vi "VI, Grow Panel Height to Control.vi"(5 "margin (20)":i32=20, 6 "error in":errorcluster, 8 "Ctl ref":refnum<vi>, 9 "VI ref":refnum<vi>) -> (0 "error out":errorcluster, 2 "Ctl ref dup":refnum<vi>, 3 "VI ref dup":refnum<vi>)   [LabVIEW 2010]
doc: "This function increases a panels width to display a control."
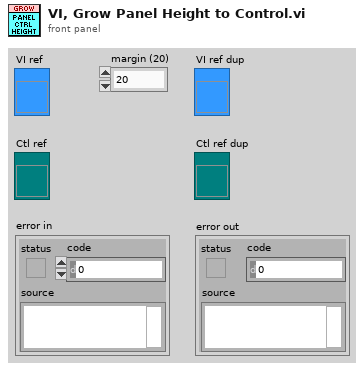
[diagram p1: front panel]
types:
  T1 = typedef "LVRectTypeDef.ctl" = cluster{"left":i16, "top":i16, "right":i16, "bottom":i16}
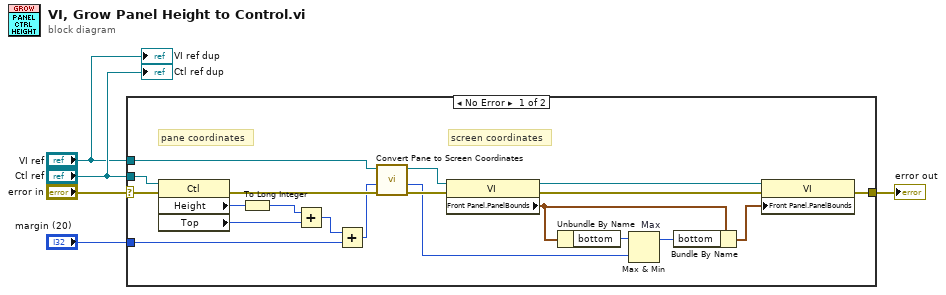
[diagram p0: block diagram]
diagram:
  n1 = case shown="No Error" "error in" {
    selector: "error in" -> [w25 w26]
    tunnel: [w21 w26] -> w5
    tunnel: "Ctl ref" -> [w6 _]
    tunnel: "VI ref" -> [w16 _]
    tunnel: "margin (20)" -> [w23 _]
    frame No Error {
      # "screen coordinates"
      # "pane coordinates"
      n2 = property class="Ctl"(reference=w6, error in=w25) -> (error out=w15:errorcluster, "Height"=w12:u32, "Top"=w11:i32)  [unwired: 1 out]
      n3 = To Long Integer(number=w12) -> (32bit integer=w10:i32)
      n4 = Add(x=w10, y=w11) -> (x+y=w18:i32)
      n5 = Add(x=w18, y=w23) -> (x+y=w9:i32)
      n6 = call "Convert Pane to Screen Coordinates.vi"("error in"=w15, "Vertical"=w9, "VI ref"=w16) -> ("error out"=w14:errorcluster, "Vertical out"=w8:i16, "VI ref dup"=w13:refnum<vi>)  [unwired: 3 in, 1 out]
      n7 = property class="VI"(reference=w13, error in=w14) -> (reference out=w20:refnum<vi>, error out=w22:errorcluster, "Front Panel.PanelBounds"=w24:T1)
      n8 = Unbundle By Name(w24) -> ("bottom"=w19:i16)
      n9 = Max & Min "Max"(x=w19, y=w8) -> (max(x,y)=w17:i16)  [unwired: 1 out]
      n10 = Bundle By Name(cluster=w24, "bottom"=w17) -> (w7:T1)
      n11 = property class="VI"(reference=w20, error in=w22, "Front Panel.PanelBounds"=w7) -> (error out=w21:errorcluster)  [unwired: 1 out]
    }
    frame Error {
    }
  }
  "error out" <- w5
  "VI ref dup" <- "VI ref"
  "Ctl ref dup" <- "Ctl ref"
